vi "Create.vi"(9 "Current":string, 10 "Input":string) -> (3 "Proto":refnum<class "Directional Keypad.lvclass">)   [LabVIEW 2020, in "Directional Keypad.lvclass"]
uses:
  Directional Keypad.lvclass
  Directional Keypad.lvclass/Directional Keypad.ctl
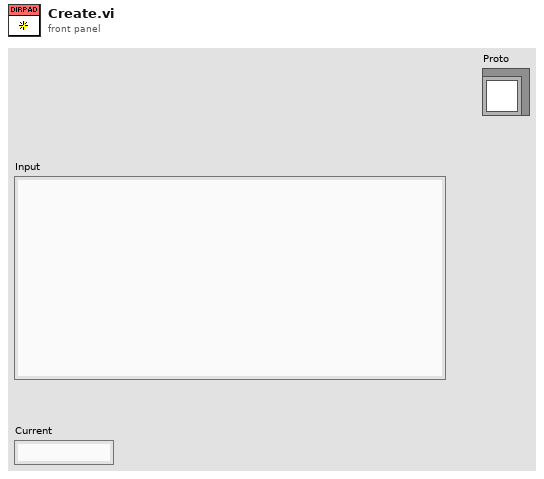
[diagram p1: front panel]
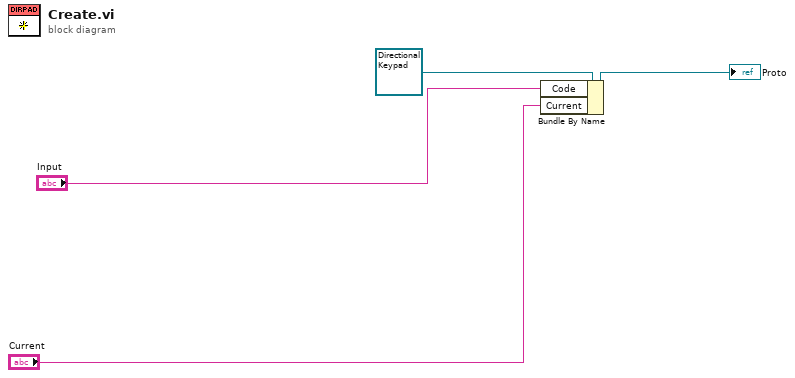
[diagram p0: block diagram]
diagram:
  n1 = Bundle By Name(cluster=refnum<class "Directional Keypad.lvclass"> refnum ("Proto"), "Code"="Input", "Current"="Current") -> (→"Proto":refnum<class "Directional Keypad.lvclass">)
